vi "末尾多余0的去处.vi"(11 "字符串":string) -> (2 "字符串 2":string)   [LabVIEW 2013]
panel:
  # "对末尾多余零的处理"
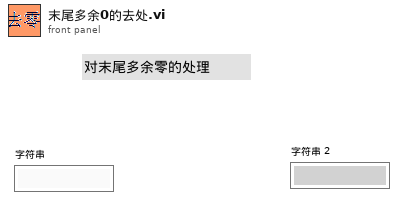
[diagram p1: front panel]
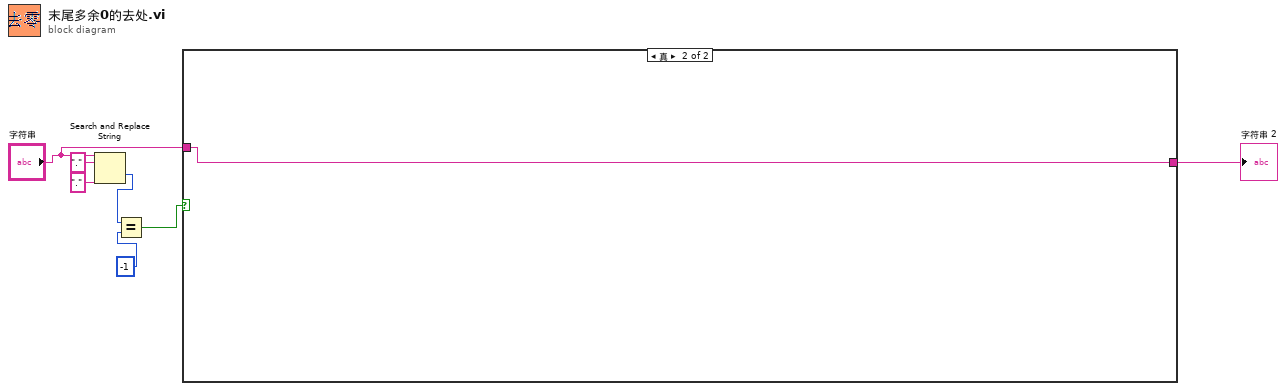
[diagram p0: block diagram]
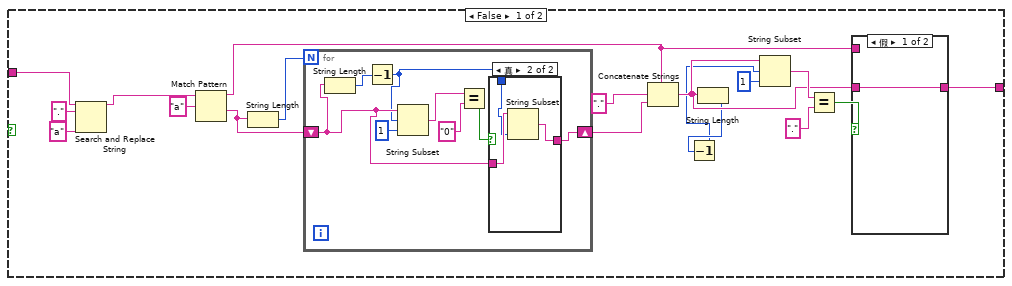
[diagram p2: hidden frame]
diagram:
  n1 = Search and Replace String(input string="字符串", search string="." ("搜索字符串"), replace string="." ("替换字符串(\"\")")) -> (offset past replacement=w5:i32)  [unwired: 5 in, 3 out]
  n2 = Equal?(x=w5, y=-1) -> (x = y?=w3:bool)
  n3 = case shown="真" w3 {
    tunnel: "字符串" -> [w24 w40]
    tunnel: [w11 w40] -> w1
    frame False {
      n4 = Search and Replace String(input string=w24, search string="." ("搜索字符串"), replace string="a" ("替换字符串(\"\")")) -> (result string=w22:string)  [unwired: 5 in, 3 out]
      n5 = Match Pattern(string=w22, regular expression="a" ("正则表达式")) -> (before substring=w12:string, after substring=w19:string)  [unwired: 1 in, 2 out]
      n6 = String Length(string=w19) -> (length=w18:i32)
      n7 = for {
        N: w18 -> [_]
        shift-right: [w29] -> w17
        shift-left: w19 -> [w30]
        n8 = String Length(string=w30) -> (length=w31:i32)
        n9 = Decrement(x=w31) -> (x-1=w28:i32)
        n10 = String Subset(string=w30, offset (0)=w28, length (rest)=1 ("长度（剩余）")) -> (substring=w33:string)
        n11 = Equal?(x=w33, y="0") -> (x = y?=w32:bool)
        n12 = case shown="真" w32 {
          tunnel: w30 -> [w36 w39]
          tunnel: [w36 w37] -> w29
          tunnel: w28 -> [_ w38]
          frame False {
          }
          frame True {
            n13 = String Subset(string=w39, length (rest)=w38) -> (substring=w37:string)  [unwired: 1 in]
          }
        }
      }
      n14 = Concatenate Strings(w12, ".", w17) -> (w10:string)
      n15 = String Length(string=w10) -> (length=w9:i32)
      n16 = Decrement(x=w9) -> (x-1=w8:i32)
      n17 = String Subset(string=w10, offset (0)=w8, length (rest)=1 ("长度（剩余）")) -> (substring=w15:string)
      n18 = Equal?(x=w15, y=".") -> (x = y?=w13:bool)
      n19 = case shown="假" w13 {
        tunnel: w12 -> [_ w27]
        tunnel: [w26 w27] -> w11
        tunnel: w10 -> [w26 _]
        frame False {
        }
        frame True {
        }
      }
    }
    frame True {
    }
  }
  "字符串 2" <- w1
